vi "Send Keyboard Data.vi"(7 "Robot IP":string, 10 "keys pressed":T1(array[ring])) -> ()   [LabVIEW 2015]
uses:
  Common Code/Keyboard Packet.ctl
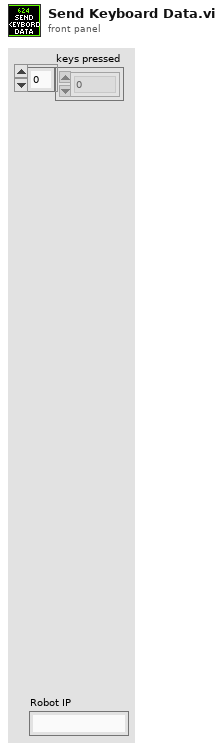
[diagram p1: front panel]
types:
  T1 = enum16{"0", "1", "2", "3", "4", "5", "6", "7", "8", "9", "A", "B", "C", "D", "E", "F", "G", "H", "I", "J", "K", "L", "M", "N", "O", "P", "Q", "R", "S", "T", "U", "V", "W", "X", "Y", "Z", "F1", "F2", "F3", "F4", "F5", "F6", "F7", "F8", "F9", "F10", "F11", "F12", "F13", "F14", "F15", "ADD", "BACK", "BACKSLASH", "CAPITAL", "COMMA", "DECIMAL", "DELETE", "DIVIDE", "DOWN", "END", "EQUALS", "ESCAPE", "GRAVE (`)", "HOME", "INSERT", "LBRACKET", "LCONTROL", "LEFT", "L ALT", "LSHIFT", "LWIN", "MINUS", "MULTIPLY", "NEXT", "NUMLOCK", "NUMPAD_0", "NUMPAD_1", "NUMPAD_2", "NUMPAD_3", "NUMPAD_4", "NUMPAD_5", "NUMPAD_6", "NUMPAD_7", "NUMPAD_8", "NUMPAD_9", "PAUSE", "PERIOD", "PRIOR (PG UP)", "RBRACKET", "RCONTROL", "RETURN", "RIGHT", "R ALT", "RSHIFT", "RWIN", "SCROLL", "SEMICOLON", "SLASH", "SPACE", "SUBTRACT", "TAB", "UP", "ENTER (num pad)", "' (quote)"}[]
  T2 = typedef "Keyboard Packet.ctl" = cluster{"keys pressed":enum16{"0", "1", "2", "3", "4", "5", "6", "7", "8", "9", "A", "B", "C", "D", "E", "F", "G", "H", "I", "J", "K", "L", "M", "N", "O", "P", "Q", "R", "S", "T", "U", "V", "W", "X", "Y", "Z", "F1", "F2", "F3", "F4", "F5", "F6", "F7", "F8", "F9", "F10", "F11", "F12", "F13", "F14", "F15", "ADD", "BACK", "BACKSLASH", "CAPITAL", "COMMA", "DECIMAL", "DELETE", "DIVIDE", "DOWN", "END", "EQUALS", "ESCAPE", "GRAVE (`)", "HOME", "INSERT", "LBRACKET", "LCONTROL", "LEFT", "L ALT", "LSHIFT", "LWIN", "MINUS", "MULTIPLY", "NEXT", "NUMLOCK", "NUMPAD_0", "NUMPAD_1", "NUMPAD_2", "NUMPAD_3", "NUMPAD_4", "NUMPAD_5", "NUMPAD_6", "NUMPAD_7", "NUMPAD_8", "NUMPAD_9", "PAUSE", "PERIOD", "PRIOR (PG UP)", "RBRACKET", "RCONTROL", "RETURN", "RIGHT", "R ALT", "RSHIFT", "RWIN", "SCROLL", "SEMICOLON", "SLASH", "SPACE", "SUBTRACT", "TAB", "UP", "ENTER (num pad)", "' (quote)"}[]}
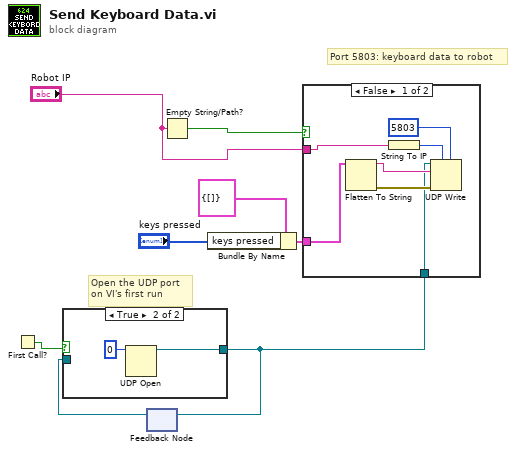
[diagram p0: block diagram]
diagram:
  # "Open the UDP port\non VI's first run"
  # "Port 5803: keyboard data to robot"
  n1 = First Call?() -> (First Call?: T/F=w5:bool)
  n2 = feedback #1() -> (w6:refnum<k16>)  [unwired: 1 in]
  n3 = case shown="True" w5 {
    tunnel: w6 -> [w9 _]
    tunnel: [w9 w10] -> w4
    frame False {
    }
    frame True {
      n4 = UDP Open(11:u16 0 ("port")) -> (port=w10:refnum<k16>)  [unwired: 4 in, 2 out]
    }
  }
  n5 = feedback-in #1(w4) -> ()
  n6 = Empty String/Path?(string/path="Robot IP") -> (empty?=w8:bool)
  n7 = Bundle By Name(cluster=T2 {"keys pressed"=[]} ("Cluster"), "keys pressed"="keys pressed") -> (w1:T2)
  n8 = case shown="False" w8 {
    tunnel: "Robot IP" -> [w18 _]
    tunnel: w4 -> [w13 _]
    tunnel: w1 -> [w12 _]
    frame False {
      n9 = Flatten To String(anything=w12) -> (data string=w16:string, error out=w17:errorcluster)  [unwired: 3 in, 1 out]
      n10 = String To IP(1:w18) -> (0:w15:u32)
      n11 = UDP Write(address=w15, port or service name=u16 5803, connection ID=w13, data in=w16, 8:w17) -> ()  [unwired: 1 in, 2 out]
    }
    frame True {
      # "The robot IP is not\nready yet, don't try\nto send data"
    }
  }
